vi "Yaw Pitch Roll.vi"(10 "R Rotation Matrix":T1 format="%#_6f") -> (1 "Roll":dbl, 2 "Pitch":dbl, 3 "Yaw":dbl)   [LabVIEW 2025]
uses:
  <vilib>/Analysis/Matrix/Datatypes/RealMatrix.ctl
  <vilib>/Analysis/Matrix/NI_Matrix.lvlib
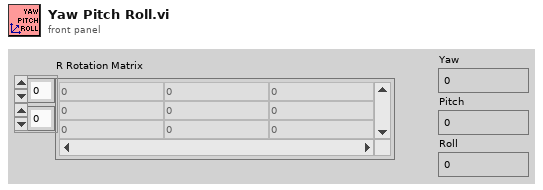
[diagram p1: front panel]
types:
  T1 = typedef "NI_Matrix.lvlib/RealMatrix.ctl" = dbl[][]
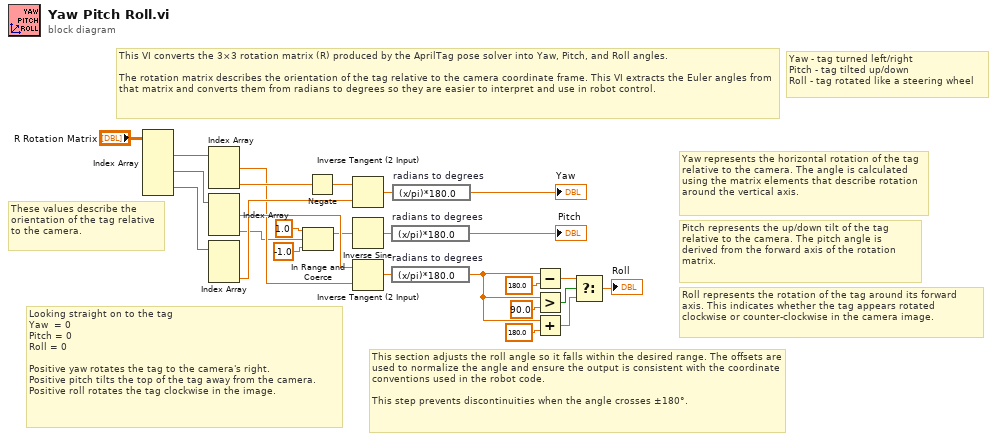
[diagram p0: block diagram]
diagram:
  # "These values describe the orientation of the tag relative to the camera."
  # "Looking straight on to the tag\nYaw  = 0\nPitch = 0\nRoll = 0\n\nPositive yaw rotates the tag to the camera's right.\nPositive pitch tilts the top of the tag away from the camera.\nPositive roll rotates the tag clockwise in the image."
  # "Yaw - tag turned left/right\nPitch - tag tilted up/down\nRoll - tag rotated like a steering wheel"
  # "This section adjusts the roll angle so it falls within the desired range. The offsets are used to normalize the angle and ensure the output is consistent with the coordinate conventions used in the robot code.\n\nThis step prevents discontinuities when the angle crosses ±180°."
  # "Roll represents the rotation of the tag around its forward axis. This indicates whether the tag appears rotated clockwise or counter-clockwise in the camera image."
  # "Pitch represents the up/down tilt of the tag relative to the camera. The pitch angle is derived from the forward axis of the rotation matrix."
  # "Yaw represents the horizontal rotation of the tag relative to the camera. The angle is calculated using the matrix elements that describe rotation around the vertical axis."
  # "This VI converts the 3×3 rotation matrix (R) produced by the AprilTag pose solver into Yaw, Pitch, and Roll angles.\n\nThe rotation matrix describes the orientation of the tag relative to the camera coordinate frame. This VI extracts the Euler angles from that matrix and converts them from radians to degrees so they are easier to interpret and use in robot control."
  n1 = Index Array(array="R Rotation Matrix") -> (element #1=w19:dbl[], element #2=w26:dbl[], element #3=w18:dbl[])  [unwired: 6 in]
  n2 = Index Array(array=w19) -> (element #1=w14:dbl, element #3=w17:dbl)  [unwired: 3 in, 1 out]
  n3 = Index Array(array=w26) -> (element #1=w23:dbl, element #3=w3:dbl)  [unwired: 3 in, 1 out]
  n4 = Index Array(array=w18) -> (element #3=w15:dbl)  [unwired: 3 in, 2 out]
  n5 = In Range and Coerce(upper limit=1.0, x=w3, lower limit=-1.0) -> (coerced(x)=w2:dbl)  [unwired: 1 out]
  n6 = Negate(x=w17) -> (-x=w16:dbl)
  n7 = Inverse Tangent (2 Input)(1:w15, 2:w16) -> (0:w21:dbl)
  n8 = Inverse Sine(1:w2) -> (0:w24:dbl)
  n9 = Inverse Tangent (2 Input)(1:w14, 2:w23) -> (0:w25:dbl)
  n10 = expression code="(x/pi)*180.0" "radians to degrees"(w24) -> (→"Pitch":dbl)
  n11 = expression code="(x/pi)*180.0" "radians to degrees"(w25) -> (w9:dbl)
  n12 = expression code="(x/pi)*180.0" "radians to degrees"(w21) -> (→"Yaw":dbl)
  n13 = Subtract(x=w9, y=180.0) -> (x-y=w7:dbl)
  n14 = Greater?(x=w9, y=90.0) -> (0:w12:bool)
  n15 = Add(x=w9, y=180.0) -> (x+y=w8:dbl)
  n16 = Select(t=w7, s=w12, f=w8) -> (s? t:f=→"Roll":dbl)
